vi "Connection Handler VI.vi"(9 "Additional Data":variant, 10 "connection ID":T1, 11 "TCP Server Refnum":refnum<class "JKI TCP Server.lvclass">) -> ()   [LabVIEW 2020]
uses:
  <vilib>/addons/_JKI.lib/_JKI_lib_TCP_Server.llb/TCP Server Connection Session ID Cluster.ctl
  <vilib>/addons/_JKI.lib/_JKI_lib_TCP_Server.llb/JKI TCP Server.lvclass
  <userlib>/_NEVSTOP/Communicable State Machine(CSM)/_Support/Priority Queue/Priority Queue.lvclass/Priority Queue.ctl
  bd168d05-2ccd-4f69-90c9-be1b4e621865.vi
  <userlib>/_NEVSTOP/Communicable State Machine(CSM)/_Support/Common/Trim Single line Text.vi
  <userlib>/_NEVSTOP/Communicable State Machine(CSM)/_Support/Process/CSMP-Sync Call.vi
  <userlib>/_NEVSTOP/Communicable State Machine(CSM)/Utility/uuid.vi
  <userlib>/_NEVSTOP/Communicable State Machine(CSM)/Utility/Build Error Cluster.vi
  <userlib>/_NEVSTOP/Communicable State Machine(CSM)/AdvanceAPI/CSM - Make String Arguments Safe.vi
  <userlib>/_NEVSTOP/Communicable State Machine(CSM)/_Support/CSMQ/_CSMObj-Message Check.vi
  <userlib>/_NEVSTOP/Communicable State Machine(CSM)/_Support/CSMQ/_CSMObj-Enqueue Cross-Module Message.vi
  <userlib>/_NEVSTOP/Communicable State Machine(CSM)/_Support/CSMQ/_CSMOFGV Get.vi
  <userlib>/_NEVSTOP/Communicable State Machine(CSM)/AdvanceAPI/CSM - Keywords.vi
  <userlib>/_NEVSTOP/Communicable State Machine(CSM)/_Support/Priority Queue/Enqueue Element.vi
  <userlib>/_NEVSTOP/Communicable State Machine(CSM)/_Support/FGV-BroadcastRegistry/global-CSMQ FGV Change Flag.vi
  <userlib>/_NEVSTOP/Communicable State Machine(CSM)/_Support/CSMQ/_CSMOFGV.vi
  <userlib>/_NEVSTOP/Communicable State Machine(CSM)/addons/API-String-Arugments-Support/_Support/Data To API String Arguments.vi
  <userlib>/_NEVSTOP/Communicable State Machine(CSM)/_Support/Message/Parse State with Arguments String.vi
  <userlib>/_NEVSTOP/Communicable State Machine(CSM)/_Support/Error/CSM No Target Error.vi
  <userlib>/_NEVSTOP/Communicable State Machine(CSM)/_Support/Error/CSM Not Allowed Message.vi
  <userlib>/_NEVSTOP/Communicable State Machine(CSM)/_Support/Error/CSM Target Error.vi
  <userlib>/_NEVSTOP/Communicable State Machine(CSM)/_Support/Error/CSM Unhandled State Error.vi
  <userlib>/_NEVSTOP/Communicable State Machine(CSM)/_Support/Error/CSM Target Timeout Error.vi
  <userlib>/_NEVSTOP/Communicable State Machine(CSM)/_Polymophic/Build Synchronous Message with Arguments.vi
  <userlib>/_NEVSTOP/Communicable State Machine(CSM)/Communicable State Machine.lvlib
  bdc9c24a-1f2c-42e6-b7bc-35ae87af1167.vi
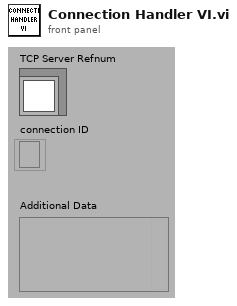
[diagram p1: front panel]
types:
  T1 = typedef "JKI TCP Server.lvclass/TCP Server Connection Session ID Cluster.ctl" = refnum<k5>
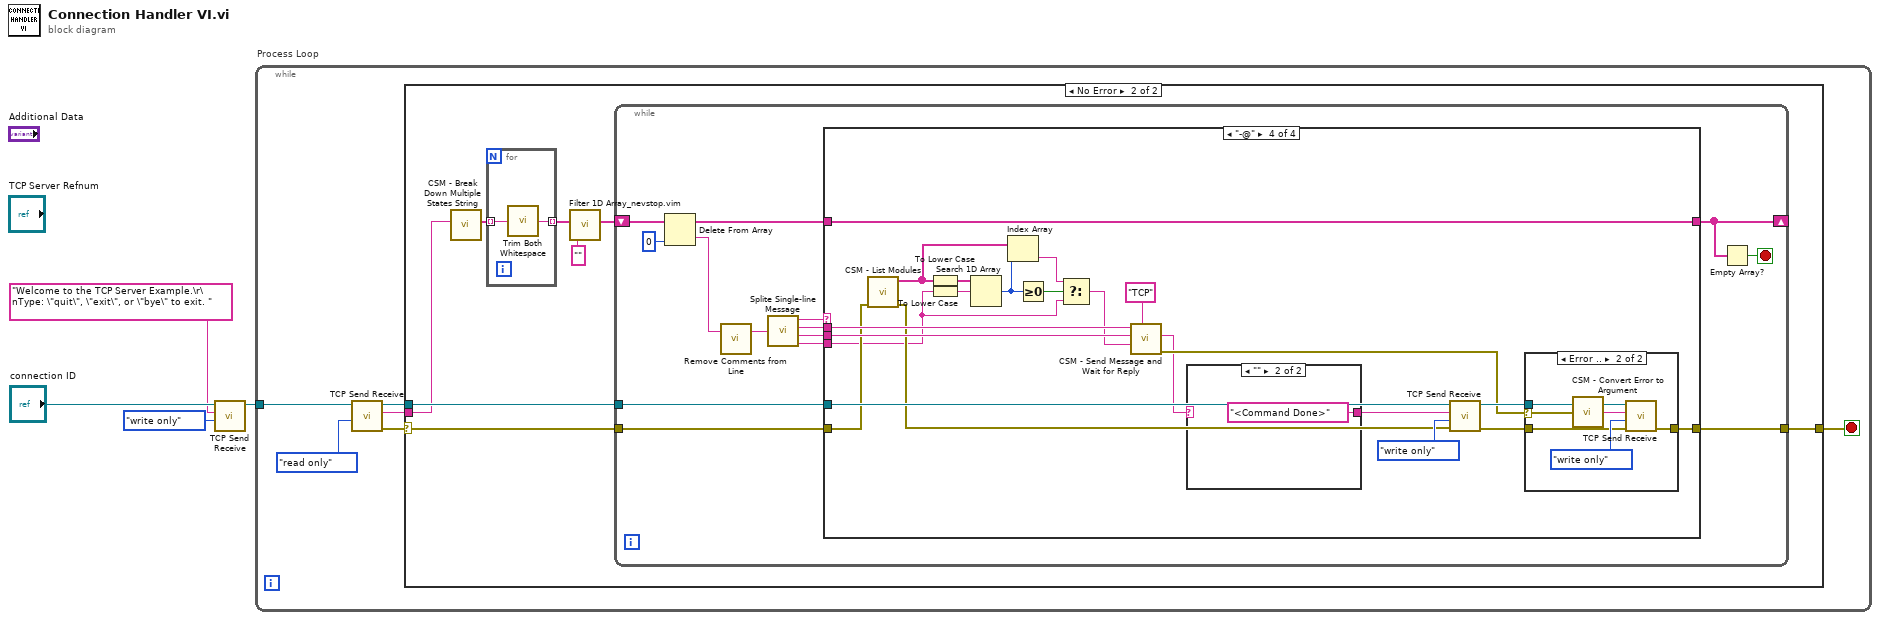
[diagram p0: block diagram]
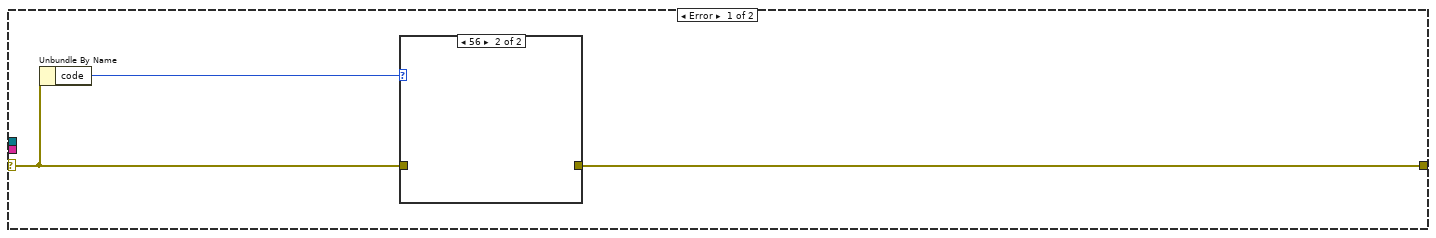
[diagram p2: hidden frame]
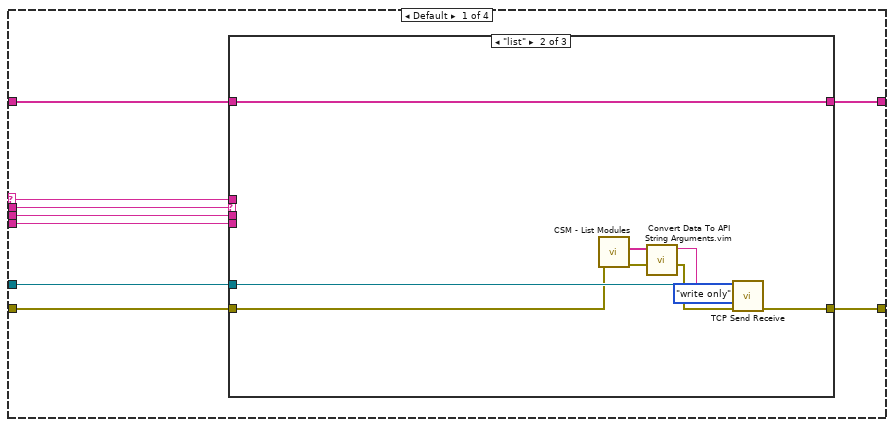
[diagram p4: hidden frame]
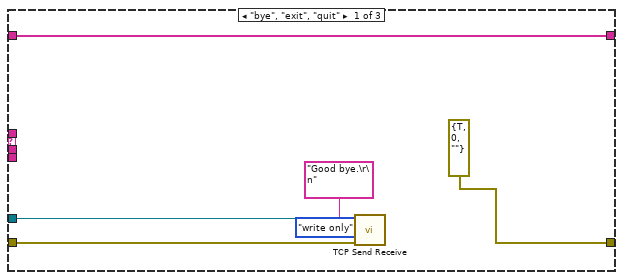
[diagram p5: hidden frame]
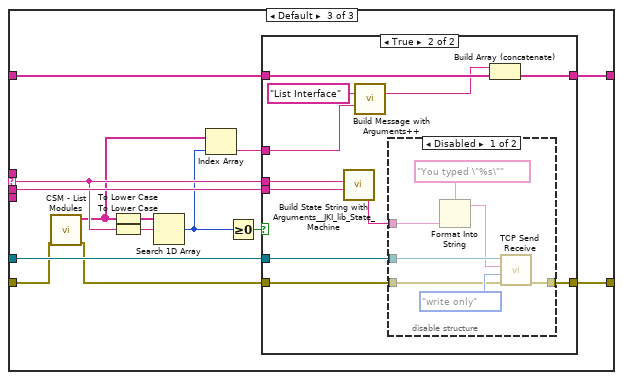
[diagram p6: hidden frame]
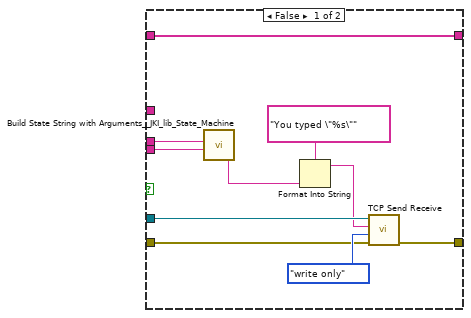
[diagram p7: hidden frame]
diagram:
  n1 = call "TCP Send Receive.vi"("access (read/write)"=enum16{"read/write", "read only", "write only"}."write only", "Data In"="Welcome to the TCP Server Example.\r\nType: \"quit\", \"exit\", or \"bye\" to exit. " ("data in"), "connection ID"="connection ID") -> ("connection ID Out"=w3:refnum<k5>)  [unwired: 6 in, 2 out]
  n2 = while "Process Loop" {
    tunnel: w3 -> [w9]
    stop <- w10 stop-if-true
    n3 = call "TCP Send Receive.vi"("access (read/write)"=enum16{"read/write", "read only", "write only"}."read only", "connection ID"=w9) -> ("error out"=w6:errorcluster, "Data Out"=w5:string, "connection ID Out"=w8:refnum<k5>)  [unwired: 7 in]
    n4 = case shown="No Error" w6 {
      selector: w6 -> [w12 w20]
      tunnel: w8 -> [_ w22]
      tunnel: w5 -> [_ w19]
      tunnel: [w11 w21] -> w10
      frame Error {
        n5 = Unbundle By Name(w12) -> ("code"=w13:i32)
        n6 = case shown="56" w13 {
          tunnel: w12 -> [w14 _]
          tunnel: [w14 _] -> w11
          frame 0, Default {
          }
          frame 56 {
          }
        }
      }
      frame No Error {
        n7 = call <userlib>:"CSM - Break Down Multiple States String.vi"("States"=w19) -> ("Multiple States"=w18:string[])  [unwired: 10 in]
        n8 = for {
          tunnel: w18 -> [w24] mode=indexing
          tunnel: [w23] -> w15 mode=indexing
          n9 = call <userlib>:"Trim Both Whitespace.vi"("string"=w24) -> ("trimmed string"=w23:string)  [unwired: 1 in]
        }
        n10 = call "Filter 1D Array_nevstop.vim"("items to filter"="", "array"=w15) -> ("filtered array"=w17:string[])  [unwired: 4 in, 1 out]
        n11 = while {
          tunnel: w22 -> [w38]
          tunnel: w20 -> [w36]
          tunnel: [w37] -> w21
          shift-right: [w25] -> _
          shift-left: w17 -> [w30]
          stop <- w26 stop-if-true
          n12 = Delete From Array(array=w30, index=0) -> (deleted portion=w28:string, array with subset deleted=w29:string[])  [unwired: 1 in]
          n13 = call <userlib>:"Remove Comments from Line.vi"("single-line text"=w28) -> ("single-line text without comments"=w35:string)  [unwired: 2 in]
          n14 = call <userlib>:"Splite Single-line Message.vi"("single-line text"=w35) -> ("operator"=w34:string, "state"=w33:string, "args"=w32:string, "source/target"=w31:string)  [unwired: 6 in]
          n15 = case shown="\"-@\"" w34 {
            selector: w34 -> [w41 _ _ _]
            tunnel: w38 -> [w47 _ _ w127]
            tunnel: [w46 w107 w109 w124] -> w37
            tunnel: w36 -> [w45 w107 w109 w116]
            tunnel: w33 -> [w44 _ _ w130]
            tunnel: w32 -> [w43 _ _ w131]
            tunnel: w31 -> [w42 _ _ w111]
            tunnel: [w40 w106 w108 w120] -> w25
            tunnel: w29 -> [w39 w106 w108 w120]
            frame Default {
              n16 = case shown="\"list\"" w44 {
                selector: w44 -> [_ _ w71]
                tunnel: w47 -> [w51 w62 w76]
                tunnel: [errorcluster {"status"=TRUE, "code"=0, "source"=""} ("error out") w55 w75] -> w46
                tunnel: w45 -> [w52 w60 w73]
                tunnel: w43 -> [_ _ w74]
                tunnel: w42 -> [_ _ _]
                tunnel: w41 -> [_ _ _]
                tunnel: [w48 w54 w67] -> w40
                tunnel: w39 -> [w48 w54 w66]
                frame "bye", "exit", "quit" {
                  n17 = call "TCP Send Receive.vi"("error in (no error)"=w52, "access (read/write)"=enum16{"read/write", "read only", "write only"}."write only", "Data In"="Good bye.\r\n" ("data in"), "connection ID"=w51) -> ()  [unwired: 5 in, 3 out]
                }
                frame "list" {
                  n18 = call <userlib>:"CSM - List Modules.vi"("Error in"=w60) -> ("Error out"=w58:errorcluster, "Module Names"=w59:string[])  [unwired: 9 in]
                  n19 = call "Convert Data To API String Arguments.vim"("error in (no error)"=w58, "data"=w59) -> ("error out"=w57:errorcluster, "String"=w56:string)  [unwired: 6 in]
                  n20 = call "TCP Send Receive.vi"("error in (no error)"=w57, "access (read/write)"=enum16{"read/write", "read only", "write only"}."write only", "Data In"=w56, "connection ID"=w62) -> ("error out"=w55:errorcluster)  [unwired: 5 in, 2 out]
                }
                frame Default {
                  n21 = call <userlib>:"CSM - List Modules.vi"("Error in"=w73) -> ("Error out"=w72:errorcluster, "Module Names"=w65:string[])  [unwired: 9 in]
                  n22 = To Lower Case(string=w65) -> (all lower case string=w70:string[])
                  n23 = To Lower Case(string=w71) -> (all lower case string=w69:string)
                  n24 = Search 1D Array(1D array=w70, element=w69) -> (index of element=w64:i32)  [unwired: 1 in]
                  n25 = Index Array(array=w65, index=w64) -> (element=w63:string)
                  n26 = Greater Or Equal To 0?(x=w64) -> (x >= 0?=w68:bool)
                  n27 = case shown="True" w68 {
                    tunnel: w76 -> [w84 w97]
                    tunnel: [w83 w96] -> w75
                    tunnel: w74 -> [w81 w95]
                    tunnel: w72 -> [w79 w93]
                    tunnel: w71 -> [w78 w90]
                    tunnel: [w77 w91] -> w67
                    tunnel: w66 -> [w77 w92]
                    tunnel: w63 -> [_ w87]
                    frame False {
                      n28 = call <vilib>:"Build State String with Arguments__JKI_lib_State_Machine.vi"("Arguments (\"\")"=w81, "State"=w78) -> ("State with Arguments"=w80:string)  [unwired: 4 in]
                      n29 = Format Into String(format string="You typed \"%s\"", w80) -> (resulting string=w82:string)  [unwired: 2 in, 1 out]
                      n30 = call "TCP Send Receive.vi"("error in (no error)"=w79, "access (read/write)"=enum16{"read/write", "read only", "write only"}."write only", "Data In"=w82, "connection ID"=w84) -> ("error out"=w83:errorcluster)  [unwired: 5 in, 2 out]
                    }
                    frame True {
                      n31 = call <vilib>:"Build State String with Arguments__JKI_lib_State_Machine.vi"("Arguments (\"\")"=w95, "State"=w90) -> ("State with Arguments"=w94:string)  [unwired: 4 in]
                      n32 = call-poly <userlib>:"Build Message with Arguments++.vi"("State with Arguments"="List Interface", "Target Module (\"\")"=w87) -> ("CSM Message String"=w88:string)  [unwired: 13 in]
                      n33 = disable-structure "Diagram Disable Structure" shown="Disabled" {
                        disable-tunnel: w97 -> [w102 _]
                        disable-tunnel: [w101 w105] -> w96
                        disable-tunnel: w94 -> [w99 _]
                        disable-tunnel: w93 -> [w98 w105]
                        frame Disabled {
                          n34 = Format Into String(format string="You typed \"%s\"", w99) -> (resulting string=w100:string)  [unwired: 2 in, 1 out]
                          n35 = call "TCP Send Receive.vi"("error in (no error)"=w98, "access (read/write)"=enum16{"read/write", "read only", "write only"}."write only", "Data In"=w100, "connection ID"=w102) -> ("error out"=w101:errorcluster)  [unwired: 5 in, 2 out]
                        }
                        frame Enabled {
                        }
                      }
                      n36 = Build Array (concatenate)(w88, w92) -> (w91:string[])
                    }
                  }
                }
              }
            }
            frame "->" {
            }
            frame "->|" {
            }
            frame "-@" {
              n37 = call <userlib>:"CSM - List Modules.vi"("Error in"=w116) -> ("Error out"=w115:errorcluster, "Module Names"=w117:string[])  [unwired: 9 in]
              n38 = To Lower Case(string=w117) -> (all lower case string=w119:string[])
              n39 = To Lower Case(string=w111) -> (all lower case string=w118:string)
              n40 = Search 1D Array(1D array=w119, element=w118) -> (index of element=w114:i32)  [unwired: 1 in]
              n41 = Index Array(array=w117, index=w114) -> (element=w112:string)
              n42 = Greater Or Equal To 0?(x=w114) -> (x >= 0?=w113:bool)
              n43 = Select(t=w112, s=w113, f=w111) -> (s? t:f=w110:string)
              n44 = call <userlib>:"CSM - Send Message and Wait for Reply.vi"("Current Module(\"\" to generate a ID)"="TCP" ("Current Module(\"\" to generate a ID)"), "Target Module"=w110, "Arguments (\"\")"=w131, "State"=w130) -> ("error out"=w123:errorcluster, "Response"=w122:string)  [unwired: 5 in, 1 out]
              n45 = case shown="\"\"" w122 {
                selector: w122 -> [w132 _]
                tunnel: [w132 "<Command Done>"] -> w121
                frame "False", Default {
                }
                frame "" {
                }
              }
              n46 = call "TCP Send Receive.vi"("error in (no error)"=w115, "access (read/write)"=enum16{"read/write", "read only", "write only"}."write only", "Data In"=w121, "connection ID"=w127) -> ("error out"=w126:errorcluster, "connection ID Out"=w125:refnum<k5>)  [unwired: 5 in, 1 out]
              n47 = case shown="Error .." w123 {
                selector: w123 -> [_ w136]
                tunnel: w126 -> [w134 w139]
                tunnel: w125 -> [_ w138]
                tunnel: [w134 w137] -> w124
                frame No Error {
                }
                frame Error {
                  n48 = call <userlib>:"CSM - Convert Error to Argument.vi"("error"=w136) -> ("Argument"=w135:string)  [unwired: 4 in]
                  n49 = call "TCP Send Receive.vi"("error in (no error)"=w139, "access (read/write)"=enum16{"read/write", "read only", "write only"}."write only", "Data In"=w135, "connection ID"=w138) -> ("error out"=w137:errorcluster)  [unwired: 5 in, 2 out]
                }
              }
            }
          }
          n50 = Empty Array?(array=w25) -> (empty?=w26:bool)
        }
      }
    }
  }
